vi "EnqueData.vi"(8 "error in (no error)":errorcluster, 9 "EnqueForClusDisp":bool, 10 "EnqueForChanDisp (T)":bool=TRUE, 11 "DataReceiver in":refnum<class "DataReceiver.lvclass">) -> (0 "error out":errorcluster, 3 "DataReceiver out":refnum<class "DataReceiver.lvclass">)   [LabVIEW 2010, in "DataReceiver.lvclass"]
uses:
  DataReceiver.lvclass
  DataReceiver.lvclass/DataReceiver.ctl
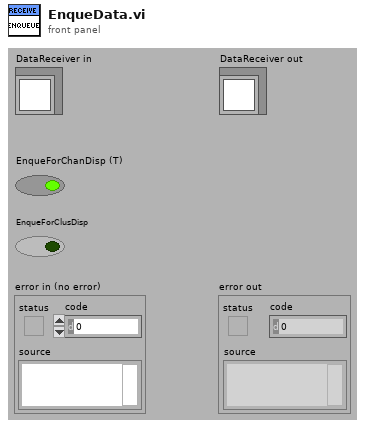
[diagram p1: front panel]
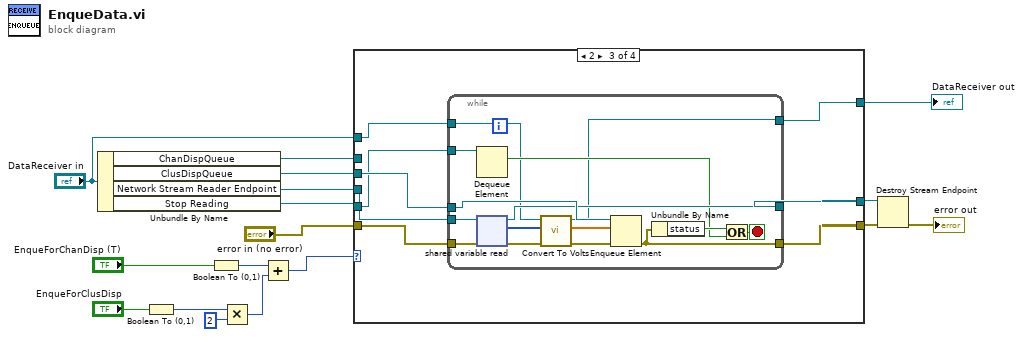
[diagram p0: block diagram]
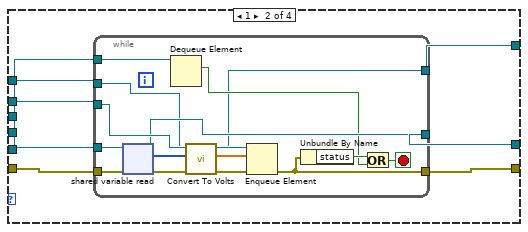
[diagram p3: hidden frame]
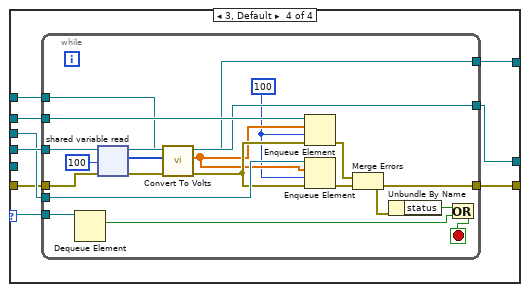
[diagram p4: hidden frame]
diagram:
  n1 = Unbundle By Name("DataReceiver in") -> ("ChanDispQueue"=w15:refnum<queue>, "ClusDispQueue"=w14:refnum<queue>, "Network Stream Reader Endpoint"=w5:refnum<k21>, "Stop Reading"=w3:refnum<queue>)
  n2 = Boolean To (0,1)(Boolean="EnqueForClusDisp") -> (0, 1=w13:i16)
  n3 = Boolean To (0,1)(Boolean="EnqueForChanDisp (T)") -> (0, 1=w11:i16)
  n4 = Multiply(x=w13, y=i16 2) -> (x*y=w10:i16)
  n5 = Add(x=w11, y=w10) -> (x+y=w9:i16)
  n6 = case shown="2" w9 {
    tunnel: w5 -> [w19 w27 w50 w75]
    tunnel: w15 -> [_ w28 _ w74]
    tunnel: w14 -> [_ _ w51 w73]
    tunnel: "error in (no error)" -> [w20 w26 w49 w72]
    tunnel: [w20 w25 w48 w71] -> w7
    tunnel: [w19 w24 w47 w70] -> w8
    tunnel: "DataReceiver in" -> [w18 w22 w45 w68]
    tunnel: w3 -> [_ w23 w46 w69]
    tunnel: [w18 w21 w44 w67] -> w1
    frame 0 {
    }
    frame 1 {
      n7 = while {
        tunnel: w27 -> [w43]
        tunnel: w28 -> [w42]
        tunnel: w26 -> [w41]
        tunnel: [w40] -> w25
        tunnel: [w39] -> w24
        tunnel: w23 -> [w36]
        tunnel: w22 -> [w32]
        tunnel: [w31] -> w21
        stop <- w37 stop-if-true
        n8 = shared-variable-read(w43, w41) -> (w39:refnum<k21>, w34:errorcluster, w30:i32[])  [unwired: 1 in, 1 out]
        n9 = Dequeue Element(queue=w36) -> (element=w35:bool)  [unwired: 2 in, 3 out]
        n10 = call-dynamic "Convert To Volts.vi"("error in (no error)"=w34, "Raw Data"=w30, "DataReceiver in"=w32) -> ("error out"=w33:errorcluster, "Volts"=w29:dbl[], "DataReceiver out"=w31:refnum<class "DataReceiver.lvclass">)  [unwired: 6 in]
        n11 = Enqueue Element(queue=w42, element=w29, error in (no error)=w33) -> (error out=w40:errorcluster)  [unwired: 1 in, 2 out]
        n12 = Unbundle By Name(w40) -> ("status"=w38:bool)
        n13 = Or(x=w38, y=w35) -> (x .or. y?=w37:bool)
      }
    }
    frame 2 {
      n14 = while {
        tunnel: w50 -> [w66]
        tunnel: w51 -> [w65]
        tunnel: w49 -> [w64]
        tunnel: [w63] -> w48
        tunnel: [w62] -> w47
        tunnel: w46 -> [w61]
        tunnel: w45 -> [w54]
        tunnel: [w53] -> w44
        stop <- w60 stop-if-true
        n15 = Dequeue Element(queue=w61) -> (element=w58:bool)  [unwired: 2 in, 3 out]
        n16 = shared-variable-read(w66, w64) -> (w62:refnum<k21>, w57:errorcluster, w55:i32[])  [unwired: 1 in, 1 out]
        n17 = call-dynamic "Convert To Volts.vi"("error in (no error)"=w57, "Raw Data"=w55, "DataReceiver in"=w54) -> ("error out"=w56:errorcluster, "Volts"=w52:dbl[], "DataReceiver out"=w53:refnum<class "DataReceiver.lvclass">)  [unwired: 6 in]
        n18 = Enqueue Element(queue=w65, element=w52, error in (no error)=w56) -> (error out=w63:errorcluster)  [unwired: 1 in, 2 out]
        n19 = Unbundle By Name(w63) -> ("status"=w59:bool)
        n20 = Or(x=w59, y=w58) -> (x .or. y?=w60:bool)
      }
    }
    frame 3, Default {
      n21 = while {
        tunnel: w75 -> [w95]
        tunnel: w74 -> [w94]
        tunnel: w73 -> [w93]
        tunnel: w72 -> [w92]
        tunnel: [w89] -> w71
        tunnel: [w88] -> w70
        tunnel: w69 -> [w86]
        tunnel: w68 -> [w80]
        tunnel: [w79] -> w67
        stop <- w84 stop-if-true
        w76 = 100 ("timeout in ms (-1)")
        n22 = Dequeue Element(queue=w86) -> (element=w87:bool)  [unwired: 2 in, 3 out]
        n23 = shared-variable-read(w95, w92, 100 ("Network Stream Read Timeout")) -> (w88:refnum<k21>, w83:errorcluster, w78:i32[])  [unwired: 1 out]
        n24 = call-dynamic "Convert To Volts.vi"("error in (no error)"=w83, "Raw Data"=w78, "DataReceiver in"=w80) -> ("error out"=w82:errorcluster, "Volts"=w77:dbl[], "DataReceiver out"=w79:refnum<class "DataReceiver.lvclass">)  [unwired: 6 in]
        n25 = Enqueue Element(queue=w94, element=w77, timeout in ms (-1)=w76, error in (no error)=w82) -> (error out=w91:errorcluster)  [unwired: 2 out]
        n26 = Enqueue Element(queue=w93, element=w77, timeout in ms (-1)=w76, error in (no error)=w82) -> (error out=w90:errorcluster)  [unwired: 2 out]
        n27 = Merge Errors(w91, w90) -> (w89:errorcluster)
        n28 = Unbundle By Name(w89) -> ("status"=w85:bool)
        n29 = Or(x=w85, y=w87) -> (x .or. y?=w84:bool)
      }
    }
  }
  "DataReceiver out" <- w1
  n30 = Destroy Stream Endpoint(8:w7, 11:w8) -> (0:→"error out":errorcluster)
